vi "Test Math.vi"(8 "error in (no error)":errorcluster) -> (0 "error out":errorcluster)   [LabVIEW 2009]
doc: "This example demonstrates how to create a test suite with multiple inner test cases."
uses:
  classes/Test/Test.lvclass
panel:
  # "See block diagram"
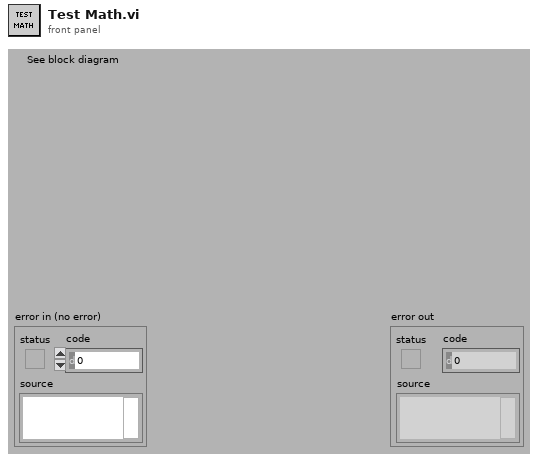
[diagram p1: front panel]
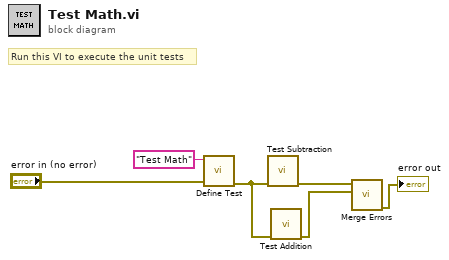
[diagram p0: block diagram]
diagram:
  # "Run this VI to execute the unit tests"
  n1 = call "Define Test.vi"("error in (no error)"="error in (no error)", "Label (VI Title)"="Test Math") -> ("error out"=w4:errorcluster)  [unwired: 9 in]
  n2 = call "Test Subtraction.vi"("error in (no error)"=w4) -> ("error out"=w2:errorcluster)  [unwired: 10 in]
  n3 = call "Test Addition.vi"("error in (no error)"=w4) -> ("error out"=w1:errorcluster)  [unwired: 10 in]
  n4 = call <vilib>:"Merge Errors.vi"("error in 2 (no error)"=w1, "error in 1 (no error)"=w2) -> ("error out"=→"error out":errorcluster)  [unwired: 5 in]
